vi "TCP_server.vi"(8 "error in (no error)":errorcluster) -> (0 "error out":errorcluster)   [LabVIEW 2023]
uses:
  enum2.ctl
  Labview/data.ctl
  Labview/commands.ctl
  <vilib>/picture/picture.llb/imagedata.ctl
panel:
  out "Input image":picture
  in  "stop":bool
  in  "Send img":bool
  in  "Load image":bool
  in  "Image path":path
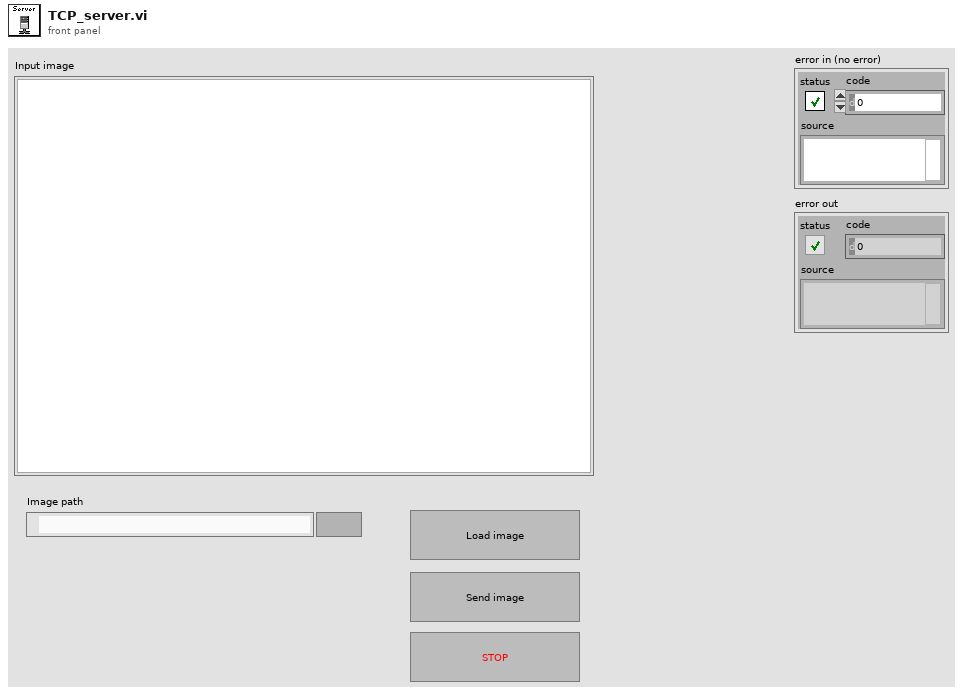
[diagram p1: front panel]
types:
  T1 = typedef "enum2.ctl" = enum16{"idle", "load", "send", "stop"}
  T2 = typedef "data.ctl" = cluster{"gui_commands":T3, "curent":T4, "ori":T4}
  T3 = typedef "commands.ctl" = enum16{"display", "bin", "gauss", "edg", "blurr", "connect", "stop", "idle"}
  T4 = typedef "imagedata.ctl" = cluster{"image type":i32, "image depth":i32, "image":u8[], "mask":u8[], "colors":u32[], "Rectangle":cluster{"left":i16, "top":i16, "right":i16, "bottom":i16}}
  T5 = typedef "LVBoundsTypeDef.ctl" = cluster{"Width":u32, "Height":u32}
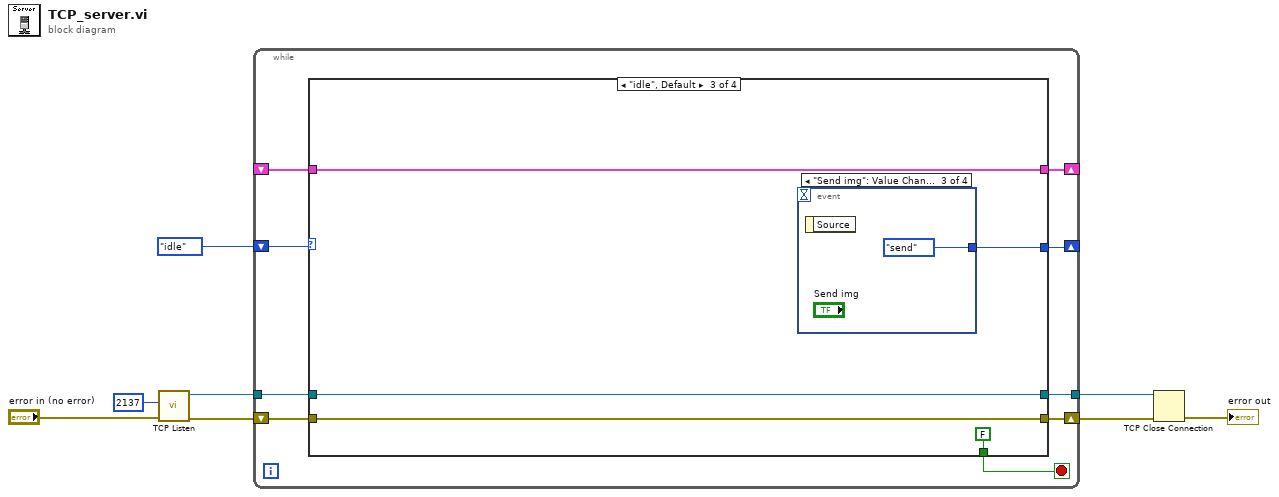
[diagram p0: block diagram]
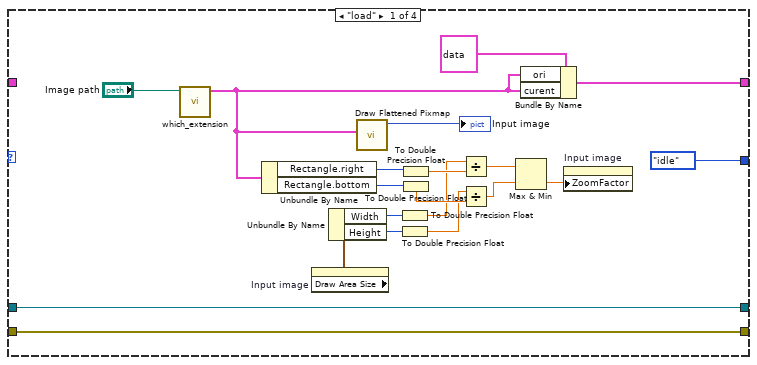
[diagram p2: hidden frame]
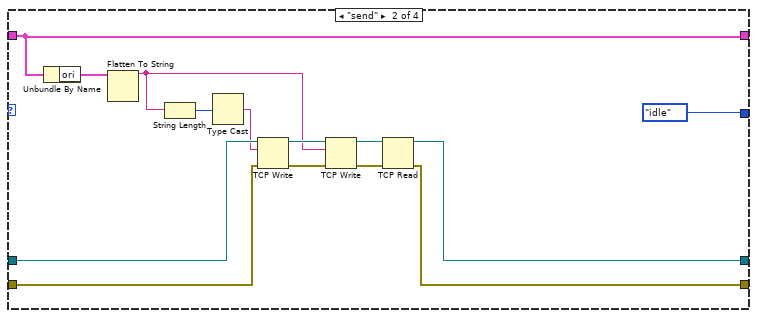
[diagram p3: hidden frame]
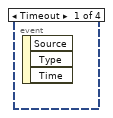
[diagram p4: hidden frame]
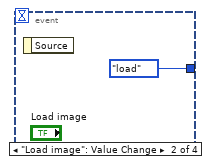
[diagram p5: hidden frame]
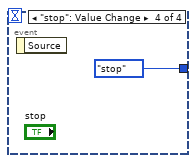
[diagram p6: hidden frame]
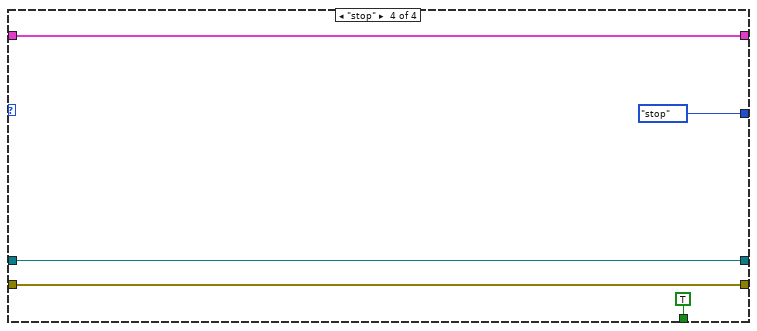
[diagram p7: hidden frame]
diagram:
  n1 = call <vilib>:"TCP Listen.vi"("error in (no error)"="error in (no error)", "port"=u16 2137) -> ("error out"=w6:errorcluster, "connection ID"=w7:refnum<k5>)  [unwired: 5 in, 3 out]
  n2 = while {
    tunnel: w7 -> [w17]
    shift-right: [w14] -> _
    shift-left: _ -> [w13]
    shift-right: [w11] -> _
    shift-left: enum2."idle" -> [w12]
    tunnel: [w10] -> w4
    shift-right: [w9] -> w3
    shift-left: w6 -> [w16]
    stop <- w15 stop-if-true
    n3 = case shown="\"idle\", Default" w12 {
      tunnel: w17 -> [w35 w51 w56 w61]
      tunnel: w16 -> [w34 w46 w55 w60]
      tunnel: [w35 w42 w56 w61] -> w10
      tunnel: [w34 w43 w55 w60] -> w9
      tunnel: [_ _ FALSE TRUE] -> w15
      tunnel: [w18 w41 w53 w63] -> w14
      tunnel: w13 -> [_ w41 w53 w63]
      tunnel: [enum2."idle" enum2."idle" w52 enum2."stop"] -> w11
      frame "load" {
        n4 = call "which_extension.vi"("Image path"="Image path") -> ("image data"=w19:T4)  [unwired: 10 in]
        n5 = Unbundle By Name(w19) -> ("Rectangle.right"=w30:i16, "Rectangle.bottom"=w31:i16)
        n6 = property on="Input image" class="Pict"() -> ("Draw Area Size"=w20:T5)  [unwired: 2 in, 2 out]
        n7 = Unbundle By Name(w20) -> ("Width"=w21:u32, "Height"=w22:u32)
        n8 = call <vilib>:"Draw Flattened Pixmap.vi"("image data"=w19) -> ("new picture"=→"Input image":picture)  [unwired: 8 in]
        n9 = To Double Precision Float(number=w21) -> (double precision float=w23:dbl)
        n10 = To Double Precision Float(number=w22) -> (double precision float=w25:dbl)
        n11 = To Double Precision Float(number=w30) -> (double precision float=w24:dbl)
        n12 = To Double Precision Float(number=w31) -> (double precision float=w26:dbl)
        n13 = Divide(x=w23, y=w24) -> (x/y=w27:dbl)
        n14 = Divide(x=w25, y=w26) -> (x/y=w28:dbl)
        n15 = Max & Min(x=w27, y=w28) -> (min(x,y)=w29:dbl)  [unwired: 1 out]
        n16 = Bundle By Name(cluster=T2 {"gui_commands"=enum."bin", "curent"={"image type"=0, "image depth"=24, "image"=array[2001000 elements], "mask"=[], "colors"=[], "Rectangle"={"left"=0, "top"=0, "right"=1000, "bottom"=667}}, "ori"={"image type"=0, "image depth"=24, "image"=array[2001000 elements], "mask"=[], "colors"=[], "Rectangle"={"left"=0, "top"=0, "right"=1000, "bottom"=667}}}, "ori"=w19, "curent"=w19) -> (w18:T2)
        n17 = property on="Input image" class="Pict"("ZoomFactor"=w29) -> ()  [unwired: 2 in, 2 out]
      }
      frame "send" {
        n18 = Unbundle By Name(w41) -> ("ori"=w39:T4)
        n19 = Flatten To String(anything=w39) -> (data string=w38:string)  [unwired: 3 in, 2 out]
        n20 = String Length(string=w38) -> (length=w50:i32)
        n21 = Type Cast(x=w50) -> (*(type *) &x=w49:string)  [unwired: 1 in]
        n22 = TCP Write(connection ID=w51, data in=w49, error in (no error)=w46) -> (connection ID out=w48:refnum<k5>, error out=w47:errorcluster)  [unwired: 1 in, 1 out]
        n23 = TCP Write(connection ID=w48, data in=w38, error in (no error)=w47) -> (connection ID out=w45:refnum<k5>, error out=w44:errorcluster)  [unwired: 1 in, 1 out]
        n24 = TCP Read(connection ID=w45, error in (no error)=w44) -> (connection ID out=w42:refnum<k5>, error out=w43:errorcluster)  [unwired: 3 in, 1 out]
      }
      frame "idle", Default {
        n25 = event shown="[2] \"Send img\": Value Change" {
          selector: _ -> [_ _ _ _]
          dyn-events: _ -> [_ _ _ _]
          timeout: _ -> [_ _ _ _]
          tunnel: [_ enum2."load" enum2."send" enum2."stop"] -> w52
          event Timeout {
            n26 = event-data() -> ()  [unwired: 1 in, 3 out]
          }
          event "Load image": Value Change {
            n27 = event-data() -> ()  [unwired: 1 in, 1 out]
          }
          event "Send img": Value Change {
            n28 = event-data() -> ()  [unwired: 1 in, 1 out]
          }
          event "stop": Value Change {
            n29 = event-data() -> ()  [unwired: 1 in, 1 out]
          }
        }
      }
      frame "stop" {
      }
    }
  }
  n30 = TCP Close Connection(connection ID=w4, error in (no error)=w3) -> (error out=→"error out":errorcluster)  [unwired: 1 in, 1 out]
